vi "Get Whale.vi"(2 "error in":errorcluster, 3 "Image":T2) -> (0 "error out":errorcluster, 1 "Matches":T1(array[cluster]) {"Bounding Box"."y" format="%.2f"; "Bounding Box"."x" format="%.2f"; "Position"."y" format="%.2f"; "Position"."x" format="%.2f"; "Score" format="%.2f"; "Scale" format="%.2f"; "Angle" format="%.2f"})   [LabVIEW 2011]
uses:
  <vilib>/vision/Image Controls.llb/IMAQ Image.ctl
panel:
  in  "ROI Descriptor":T3={"Global Rectangle"=[127, 50, 551, 422], "Contours"=[{"ID"=enum."External", "Type"=12, "Coordinates"=[127, 50, 551, 422, 0]}]} {"Contours"."Type" items=["No Selection", "Point", "Line", "Rectangle", "Oval", "Polygon", "Freehand Region", "Annulus", "Unused2", "Unused3", "Broken Line", "Freehand Line", "Rotated Rectangle"]}
  out "Templete Image":T2(plugin-control)
  in  "Location\nTemplete":path=path "C:/Users/GARLAND/Documents/Projects/Robotics I/Robotics I 3390 2012/Final project/Labview/Pool navigation/whale templete.png"
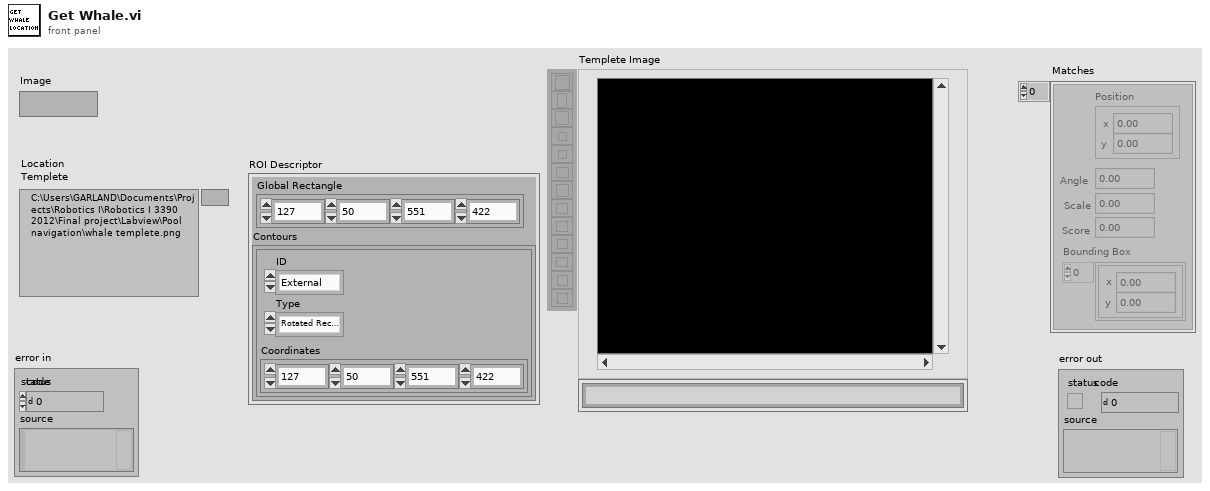
[diagram p1: front panel]
types:
  T1 = cluster{"Position":cluster{"x":sgl, "y":sgl}, "Angle":sgl, "Scale":sgl, "Score":sgl, "Bounding Box":cluster{"x":sgl, "y":sgl}[]}[]
  T2 = typedef "IMAQ Image.ctl" = refnum<image>
  T3 = cluster{"Global Rectangle":i32[], "Contours":cluster{"ID":enum32{"External", "Internal"}, "Type":u32, "Coordinates":i32[]}[]}
  T4 = typedef "Image Type" = u32
  T5 = cluster{"ROI Descriptor":cluster{"Global Rectangle":i32[], "Contours":cluster{"ID":enum32{"External", "Internal"}, "Type":u32, "Coordinates":i32[]}[]}, "Number of Matches Requested":i32, "Minimum Match Score":sgl}
  T6 = cluster{"Match Mode":u16, "Subpixel Accuracy":bool, "Rotation Angle Ranges (degrees)":cluster{sgl, sgl}[]}
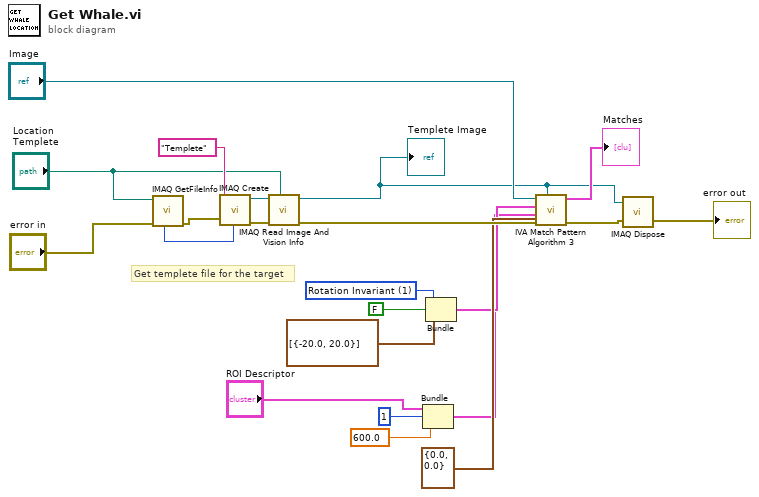
[diagram p0: block diagram]
diagram:
  w14 = u16 1 items=["Shift Invariant", "Rotation Invariant"] ("Match Mode")
  # "Get templete file for the target"
  n1 = call "IMAQ GetFileInfo"("error in (no error)"="error in", "File Path"="Location\nTemplete") -> ("error out"=w20:errorcluster, "Image Type"=w19:T4)  [unwired: 3 in, 5 out]
  n2 = call "IMAQ Create"("Image Name"="Templete", "Image Type"=w19, "error in (no error)"=w20) -> ("New Image"=w22:T2, "error out"=w21:errorcluster)  [unwired: 1 in, 1 out]
  n3 = call "IMAQ Read Image And Vision Info"("File Path"="Location\nTemplete", "error in (no error)"=w21, "Image"=w22) -> ("error out"=w11:errorcluster, "Image Out"=w1:T2)  [unwired: 1 in, 6 out]
  "Templete Image" <- w1
  n4 = Bundle("ROI Descriptor"="ROI Descriptor", "Number of Matches Requested"=1, "Minimum Match Score"=sgl 600.0) -> (w7:T5)  [unwired: 1 out]
  n5 = Bundle("Match Mode"=w14, "Subpixel Accuracy"=FALSE, "Rotation Angle Ranges (degrees)"=cluster{sgl, sgl}[] [{-20.0, 20.0}]) -> (w8:T6)  [unwired: 1 out]
  n6 = call <vilib>:"IVA Match Pattern Algorithm 3.vi"("Match Offset"=cluster{"X":sgl, "Y":sgl} {"X"=0.0, "Y"=0.0}, "Image Template"=w1, "error in (no error)"=w11, "Match Parameters"=w7, "Setup Match Parameters"=w8, "Image"="Image") -> ("error out"=w3:errorcluster, "Matches"=→"Matches":T1)  [unwired: 4 out]
  n7 = call "IMAQ Dispose"("Image"=w1, "error in (no error)"=w3) -> ("error out"=→"error out":errorcluster)  [unwired: 4 in]
